vi "Get Max Simple Profile Size.vi"() -> (1 "Max Simple Profile Size":u32)   [LabVIEW 2010, in "KEYENCE LJ-X8000A.lvlib"]
uses:
  KEYENCE LJ-X8000A.lvlib
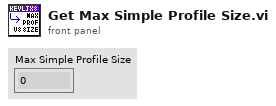
[diagram p1: front panel]
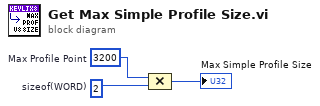
[diagram p0: block diagram]
diagram:
  w2 = u32 2  # sizeof(WORD)
  w3 = u16 3200  # Max Profile Point
  n1 = Compound Arithmetic op=MULTIPLY(w3, w2) -> (→"Max Simple Profile Size":u32)
